vi "get IR test parameters.vi"(8 "error in (no error)":errorcluster, 10 "Step":T1=1 min=1 max=99 step=1, 11 "VISA Refnum in":refnum<visa-resource-name>) -> (0 "error out":errorcluster, 3 "VISA Refnum out":refnum<visa-resource-name>, 5 "IR Parameters":T2 {"Voltage Level [V]" min=50 max=1000 step=1 format="%.3p"; "Hi Limit [ohm]" min=0.0 max=50000000000000.0 step=100000.0 format="%.1p"; "Test Time [s]" min=0.0 max=999.0 step=0.1 format="%.1p"; "Dwell Time [s]" min=0.0 max=999.0 step=0.1 format="%.1p"; "Lo Limit [ohm]" min=100000.0 max=50000000000000.0 step=100000.0 format="%.1p"; "Ramp Time [s]" min=0.0 max=999.0 step=0.1 format="%.1p"; "Fall Time [s]" min=0.0 max=999.0 step=0.1 format="%.1p"})   [LabVIEW 2025]
uses:
  IR parameters--cluster.ctl
  <instrlib>/Chroma 19052/Public/Utility/Type Def/steps--numeric.ctl
  <instrlib>/Chroma 19052/Public/Utility/Type Def/AC-DC-IR modes--ring.ctl
  <instrlib>/Chroma 19052/Public/Utility/Type Def/DC-IR modes--ring.ctl
  <instrlib>/Chroma 19052/Chroma 19052.lvlib
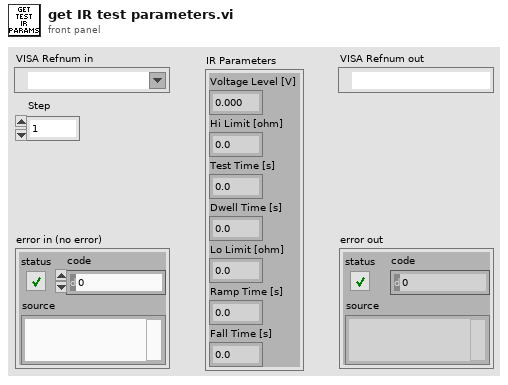
[diagram p1: front panel]
types:
  T1 = typedef "Chroma 19052.lvlib/steps--numeric.ctl" = u8
  T2 = typedef "IR parameters--cluster.ctl" = cluster{"Voltage Level [V]":u16, "Hi Limit [ohm]":dbl, "Test Time [s] ":dbl, "Dwell Time [s]":dbl, "Lo Limit [ohm]":dbl, "Ramp Time [s] ":dbl, "Fall Time [s]":dbl}
  T3 = typedef "DC-IR modes--ring.ctl" = u16
  T4 = typedef "AC-DC-IR modes--ring.ctl" = u16
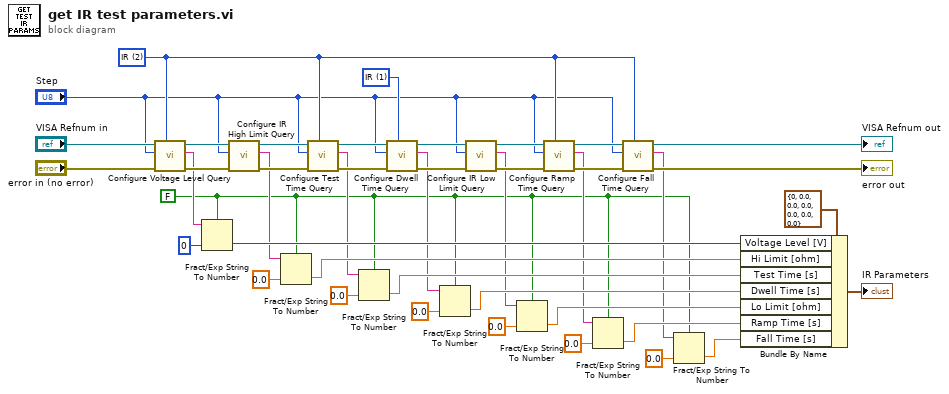
[diagram p0: block diagram]
diagram:
  w2 = FALSE ("use system decimal point (T)")
  w27 = T3 1 items=["DC", "IR"] ("Mode")
  w26 = T4 2 items=["AC", "DC", "IR"] ("Mode")
  n1 = call <instrlib>:"Configure Voltage Level Query.vi"("Mode"=w26, "error in (no error)"="error in (no error)", "Step"="Step", "VISA resource name"="VISA Refnum in") -> ("error out"=w34:errorcluster, "Voltage value [V]"=w23:string, "VISA resource name out"=w31:refnum<visa-resource-name>)  [unwired: 5 in]
  n2 = Fract/Exp String To Number(use system decimal point (T)=w2, string=w23, default (0 dbl)=u16 0 ("Voltage Level [V]")) -> (number=w21:u16)  [unwired: 1 in, 1 out]
  n3 = call <instrlib>:"Configure IR High Limit Query.vi"("error in (no error)"=w34, "Step"="Step", "VISA resource name"=w31) -> ("error out"=w37:errorcluster, "IR Hi limit value [ohm]"=w19:string, "VISA resource name out"=w38:refnum<visa-resource-name>)  [unwired: 6 in]
  n4 = Fract/Exp String To Number(use system decimal point (T)=w2, string=w19, default (0 dbl)=0.0 ("Voltage Level [V]")) -> (number=w18:dbl)  [unwired: 1 in, 1 out]
  n5 = call <instrlib>:"Configure Test Time Query.vi"("Mode"=w26, "error in (no error)"=w37, "Step"="Step", "VISA resource name"=w38) -> ("error out"=w40:errorcluster, "Test Time value [s]"=w16:string, "VISA resource name out"=w28:refnum<visa-resource-name>)  [unwired: 5 in]
  n6 = Fract/Exp String To Number(use system decimal point (T)=w2, string=w16, default (0 dbl)=0.0 ("Voltage Level [V]")) -> (number=w15:dbl)  [unwired: 1 in, 1 out]
  n7 = call <instrlib>:"Configure Dwell Time Query.vi"("Mode"=w27, "error in (no error)"=w40, "Step"="Step", "VISA resource name"=w28) -> ("error out"=w39:errorcluster, "Dwell time value [s]"=w13:string, "VISA resource name out"=w41:refnum<visa-resource-name>)  [unwired: 5 in]
  n8 = Fract/Exp String To Number(use system decimal point (T)=w2, string=w13, default (0 dbl)=0.0 ("Voltage Level [V]")) -> (number=w12:dbl)  [unwired: 1 in, 1 out]
  n9 = call <instrlib>:"Configure IR Low Limit Query.vi"("error in (no error)"=w39, "Step"="Step", "VISA resource name"=w41) -> ("error out"=w43:errorcluster, "IR Lo limit value [ohm]"=w10:string, "VISA resource name out"=w42:refnum<visa-resource-name>)  [unwired: 6 in]
  n10 = Fract/Exp String To Number(use system decimal point (T)=w2, string=w10, default (0 dbl)=0.0 ("Voltage Level [V]")) -> (number=w9:dbl)  [unwired: 1 in, 1 out]
  n11 = call <instrlib>:"Configure Ramp Time Query.vi"("Mode"=w26, "error in (no error)"=w43, "Step"="Step", "VISA resource name"=w42) -> ("error out"=w35:errorcluster, "Ramp Time value [s]"=w7:string, "VISA resource name out"=w36:refnum<visa-resource-name>)  [unwired: 5 in]
  n12 = Fract/Exp String To Number(use system decimal point (T)=w2, string=w7, default (0 dbl)=0.0 ("Voltage Level [V]")) -> (number=w6:dbl)  [unwired: 1 in, 1 out]
  n13 = call <instrlib>:"Configure Fall Time Query.vi"("Mode"=w26, "error in (no error)"=w35, "Step"="Step", "VISA resource name"=w36) -> ("error out"=→"error out":errorcluster, "Fall Time value"=w4:string, "VISA resource name out"=→"VISA Refnum out":refnum<visa-resource-name>)  [unwired: 5 in]
  n14 = Fract/Exp String To Number(use system decimal point (T)=w2, string=w4, default (0 dbl)=0.0 ("Voltage Level [V]")) -> (number=w3:dbl)  [unwired: 1 in, 1 out]
  n15 = Bundle By Name(cluster=T2 {"Voltage Level [V]"=0, "Hi Limit [ohm]"=0.0, "Test Time [s] "=0.0, "Dwell Time [s]"=0.0, "Lo Limit [ohm]"=0.0, "Ramp Time [s] "=0.0, "Fall Time [s]"=0.0} ("IR Parameters"), "Voltage Level [V]"=w21, "Hi Limit [ohm]"=w18, "Test Time [s]"=w15, "Dwell Time [s]"=w12, "Lo Limit [ohm]"=w9, "Ramp Time [s]"=w6, "Fall Time [s]"=w3) -> (→"IR Parameters":T2)
